vi "Select_Cam - コピー.vi"(8 "カメラ 3":dbl, 9 "カメラ 2":dbl, 10 "カメラ":dbl, 11 "カメラ名":string) -> (3 "出力":dbl)   [LabVIEW 2015]
panel:
  in  "ブール 3":bool
  out "ブール 2":bool
  out "ブール":bool
  out "カメラ 4":dbl
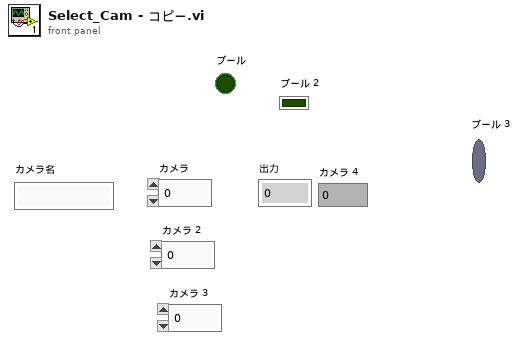
[diagram p1: front panel]
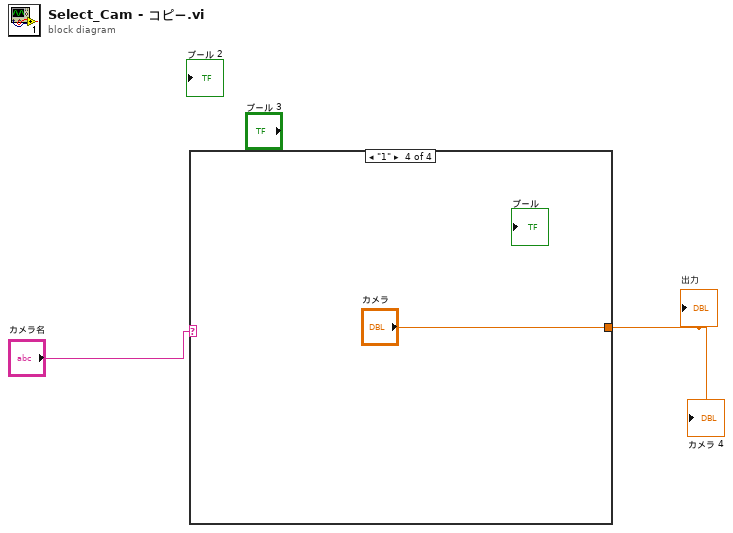
[diagram p0: block diagram]
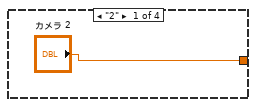
[diagram p2: hidden frame]
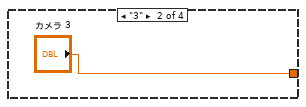
[diagram p3: hidden frame]
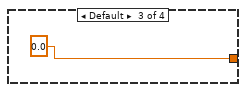
[diagram p4: hidden frame]
diagram:
  n1 = case shown="\"1\"" "カメラ名" {
    tunnel: ["カメラ 2" "カメラ 3" 0.0 "カメラ"] -> w1
    frame "2" {
    }
    frame "3" {
    }
    frame Default {
    }
    frame "1" {
    }
  }
  "出力" <- w1
  "カメラ 4" <- w1
